vi "Get Parameter Names.vi"(8 "error in (no error)":errorcluster, 11 "TDCManager":T1) -> (0 "error out":errorcluster, 2 "Parameter Names":string[](array[string]), 3 "TDCManager":T1)   [LabVIEW 2016, in "HPTDC Driver Library.lvlib"]
uses:
  HPTDC Driver Library.lvlib
  Typedefs/TDCManager.ctl
  C:/Users/CRT Controller/CRTC Labview Application/Source/HPTDC Driver Library Folder/Library files/hptdc_net4_3.7.0_x64.dll
  hptdc_net4_3.7.0_x64.dll
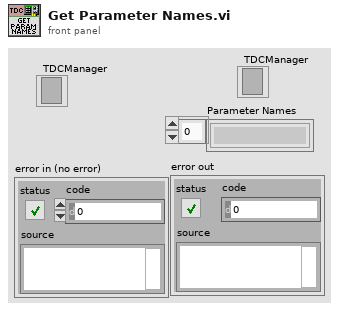
[diagram p1: front panel]
types:
  T1 = typedef "HPTDC Driver Library.lvlib/TDCManager.ctl" = refnum<k24>
  T2 = typedef "Semaphore RefNum" = refnum<k1>
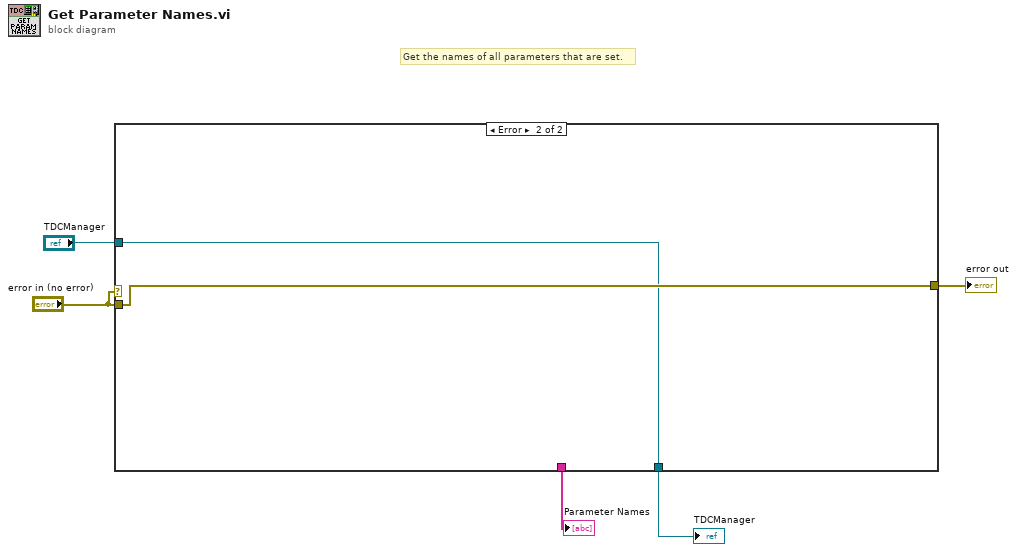
[diagram p0: block diagram]
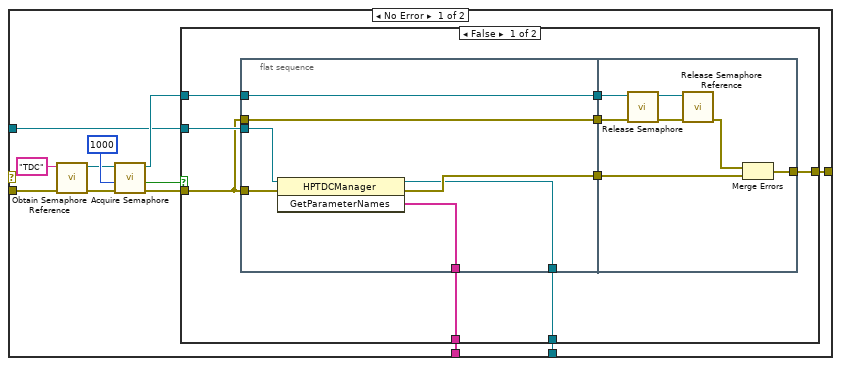
[diagram p2: hidden frame]
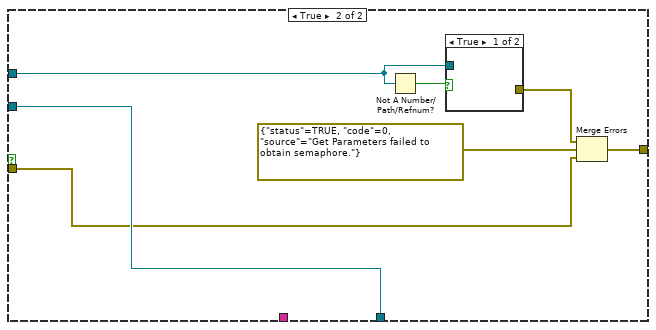
[diagram p3: hidden frame]
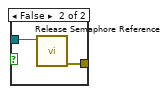
[diagram p4: hidden frame]
diagram:
  # "Get the names of all parameters that are set."
  n1 = case shown="Error" "error in (no error)" {
    tunnel: "error in (no error)" -> [w10 w51]
    tunnel: "TDCManager" -> [w9 w50]
    tunnel: [w8 w50] -> w4
    tunnel: [w7 _] -> w3
    tunnel: [w6 w51] -> w2
    frame No Error {
      n2 = call <vilib>:"Obtain Semaphore Reference.vi"("error in (no error)"=w10, "name (unnamed)"="TDC") -> ("error out"=w15:errorcluster, "semaphore"=w16:T2)  [unwired: 3 in, 1 out]
      n3 = call <vilib>:"Acquire Semaphore.vi"("error in (no error)"=w15, "ms timeout (-1)"=1000, "semaphore"=w16) -> ("error out"=w12:errorcluster, "timed out"=w13:bool, "semaphore out"=w11:T2)  [unwired: 2 in]
      n4 = case shown="False" w13 {
        tunnel: w9 -> [w26 w47]
        tunnel: w12 -> [w23 w41]
        tunnel: w11 -> [w21 w43]
        tunnel: [w20 w47] -> w8
        tunnel: [w19 w45] -> w6
        tunnel: [w18 _] -> w7
        frame False {
          n5 = flat-sequence {
            tunnel: w23 -> [w33]
            tunnel: w26 -> [w32]
            tunnel: [w31] -> w25
            tunnel: w23 -> [w30]
            tunnel: [w30] -> w24
            tunnel: [w29] -> w22
            tunnel: w21 -> [w29]
            tunnel: [w28] -> w20
            tunnel: [w27] -> w18
            tunnel: w25 -> [w40]
            tunnel: w24 -> [w37]
            tunnel: w22 -> [w35]
            tunnel: [w34] -> w19
            frame #0 {
              n6 = invoke class="HPTDCManager" method="GetParameterNames"(reference=w32, error in=w33) -> (reference out=w28:T1, error out=w31:errorcluster, "GetParameterNames"=w27:string[])  [unwired: 1 in]
            }
            frame #1 {
              n7 = call <vilib>:"Release Semaphore.vi"("error in (no error)"=w37, "semaphore"=w35) -> ("error out"=w38:errorcluster, "semaphore out"=w39:T2)  [unwired: 4 in]
              n8 = call <vilib>:"Release Semaphore Reference.vi"("error in (no error)"=w38, "semaphore"=w39) -> ("error out"=w36:errorcluster)  [unwired: 8 in, 1 out]
              n9 = Merge Errors(w36, w40) -> (w34:errorcluster)
            }
          }
        }
        frame True {
          n10 = Not A Number/Path/Refnum?(number/path/refnum=w43) -> (NaN/Path/Refnum?=w42:bool)
          n11 = case shown="True" w42 {
            tunnel: [_ w49] -> w44
            tunnel: w43 -> [_ w48]
            frame True {
            }
            frame False {
              n12 = call <vilib>:"Release Semaphore Reference.vi"("semaphore"=w48) -> ("error out"=w49:errorcluster)  [unwired: 9 in, 1 out]
            }
          }
          n13 = Merge Errors(w44, errorcluster {"status"=TRUE, "code"=0, "source"="Get Parameters failed to obtain semaphore."} ("error out"), w41) -> (w45:errorcluster)
        }
      }
    }
    frame Error {
    }
  }
  "error out" <- w2
  "TDCManager" <- w4
  "Parameter Names" <- w3
